vi "Class Name.vi"() -> (3 "class name":string)   [LabVIEW 2017, in "DSF Core.lvlib" / "Thread Interface.lvclass"]
uses:
  Thread Interface.lvclass
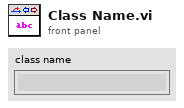
[diagram p1: front panel]
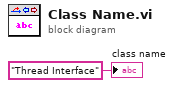
[diagram p0: block diagram]
diagram:
  "class name" <- "Thread Interface" ("class name")
